vi "TestPanel - Stage Status (eFGV).vi"(7 "Action":T1, 8 "error in":errorcluster, 11 "Stage":string[][](array[string])) -> (0 "error out":errorcluster, 2 "Stage ref":refnum<user-event>, 3 "Stage out":string[][](array[string]))   [LabVIEW 2019]
uses:
  Controls/eFGV States.ctl
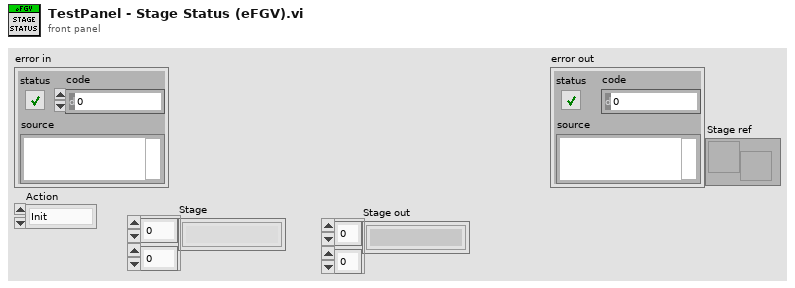
[diagram p1: front panel]
types:
  T1 = typedef "eFGV States.ctl" = enum16{"Init", "Read", "Write", "Exit"}
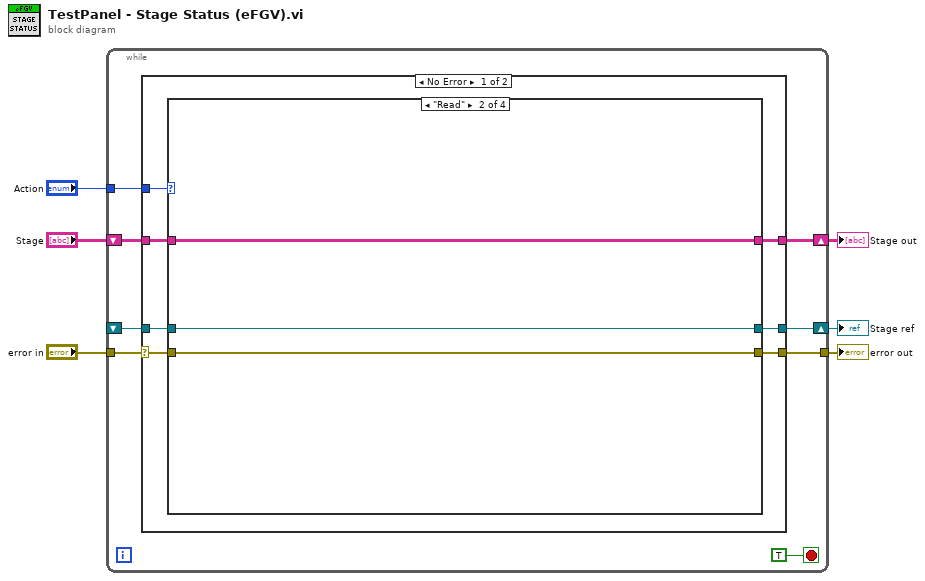
[diagram p0: block diagram]
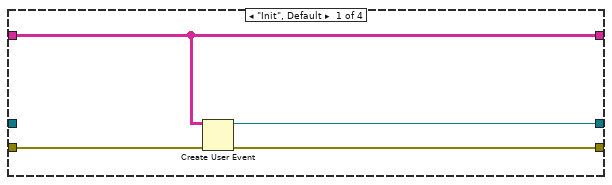
[diagram p2: hidden frame]
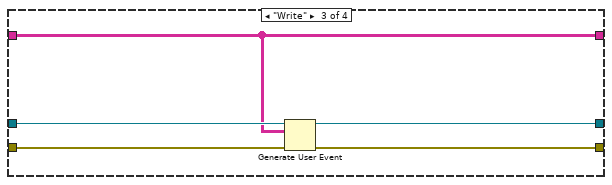
[diagram p3: hidden frame]
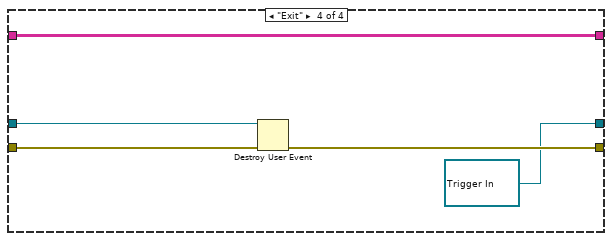
[diagram p4: hidden frame]
diagram:
  n1 = while {
    tunnel: "error in" -> [w13]
    tunnel: [w12] -> w5
    tunnel: "Action" -> [w11]
    shift-right: [w9] -> w2
    shift-left: "Stage" -> [w10]
    shift-right: [w8] -> w1
    shift-left: _ -> [w7]
    stop <- TRUE stop-if-true
    n2 = case shown="No Error" w13 {
      selector: w13 -> [w20 w41]
      tunnel: [w21 w41] -> w12
      tunnel: w11 -> [w19 _]
      tunnel: w10 -> [w18 w40]
      tunnel: [w17 w40] -> w9
      tunnel: w7 -> [w16 w39]
      tunnel: [w15 w39] -> w8
      frame No Error {
        n3 = case shown="\"Read\"" w19 {
          tunnel: [w24 w28 w33 w38] -> w21
          tunnel: w20 -> [w25 w28 w30 w37]
          tunnel: w18 -> [w23 w27 w31 w35]
          tunnel: [w23 w27 w31 w35] -> w17
          tunnel: w16 -> [_ w26 w32 w36]
          tunnel: [w22 w26 w29 refnum<user-event> refnum ("Stage")] -> w15
          frame "Init", Default {
            n4 = Create User Event(user event datatype=w23, error in=w25) -> (user event=w22:refnum<user-event>, error out=w24:errorcluster)
          }
          frame "Read" {
          }
          frame "Write" {
            n5 = Generate User Event(user event=w32, event data cluster=w31, error in=w30) -> (user event out=w29:refnum<user-event>, error out=w33:errorcluster)  [unwired: 1 in]
          }
          frame "Exit" {
            n6 = Destroy User Event(user event=w36, error in=w37) -> (error out=w38:errorcluster)
          }
        }
      }
      frame Error {
      }
    }
  }
  "error out" <- w5
  "Stage out" <- w2
  "Stage ref" <- w1
